vi "UI_WindowFrame.vi"(8 "error in (no error)":errorcluster, 11 "WindowFrame in":refnum<class "WindowFrame.lvclass">) -> (0 "error out":errorcluster, 3 "WindowFrame out":refnum<class "WindowFrame.lvclass">)   [LabVIEW 2025, in "WindowFrame.lvlib" / "WindowFrame.lvclass"]
uses:
  WindowFrame.lvclass
  C:/GitHub/danyallard/ClassUtilities/src/ClassByRef/ClassByRef.lvclass
  ClassUtilities/src/ClassByRef/ClassByRef.lvclass/ClassByRef.ctl
  <vilib>/event_ctls.llb/usereventprio.ctl
  Action.ctl
  <vilib>/Utility/miscctls.llb/LVPointTypeDef.ctl
  <vilib>/Utility/miscctls.llb/LVRectTypeDef.ctl
  FrontPanel.Open.ctl
  FrontPanel.Run-TimePosition.Centered.ctl
  FrontPanel.Run-TimePosition.Custom.ctl
  FrontPanel.Run-TimePosition.GetPosition.ctl
  SubPanelInfo.ctl
  <vilib>/Utility/miscctls.llb/LVPositionTypeDef.ctl
  <vilib>/Utility/miscctls.llb/LVBoundsTypeDef.ctl
  947dc2d2-893a-4bb1-96e4-45aff6c94e7a.vi
  ClassUtilities/src/ClassByRef/GetExitEvent.vi
  ClassUtilities/src/ClassByRef/GetNotifier.vi
  ClassUtilities/src/ClassByRef/GetExitEvent.vi/d78f5ac1-b881-48f7-a86d-8a9fda2b8e49.vi
  ClassUtilities/src/ClassByRef/GetNotifier.vi/815770e3-f244-4544-877a-43bf45f14863.vi
  ClassUtilities/src/ClassByRef/GetRef.vi
  GetEventActionRef.vi
  GetEventCloseRef.vi
  GetEventStateRef.vi
  ClassUtilities/src/ClassByRef/ClassByRef.lvclass
panel:
  in  "Close":bool
  in  "Maximize":bool
  in  "Minimize":bool
  out "TitleBar":bool=TRUE
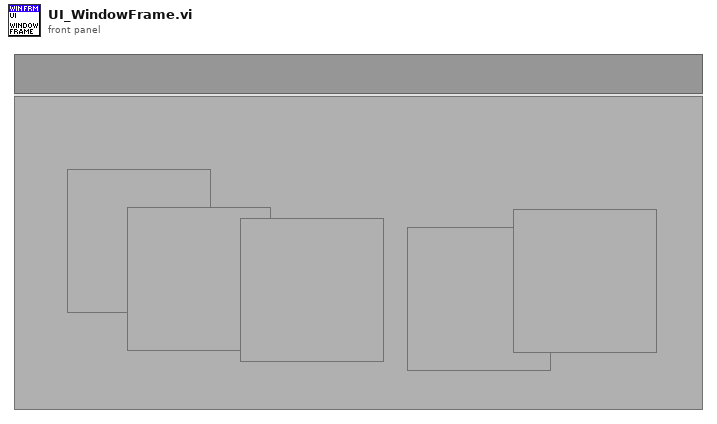
[diagram p1: front panel]
types:
  T1 = typedef "usereventprio.ctl" = enum32{"high priority", "normal priority"}
  T2 = enum32{"Invalid", "Standard", "Closed", "Hidden", "Minimized", "Maximized"}
  T3 = enum32{"Invalid", "Default", "Floating", "Floating/Auto-Hide", "Modal"}
  T4 = enum8{"Enabled", "Disabled", "Disabled and Grayed Out"}
  T5 = typedef "LVPointTypeDef.ctl" = cluster{"Horizontal":i16, "Vertical":i16}
  T6 = typedef "LVRectTypeDef.ctl" = cluster{"Left":i16, "Top":i16, "Right":i16, "Bottom":i16}
  T7 = typedef "WindowFrame.lvlib/WindowFrame.lvclass/FrontPanel.Open.ctl" = cluster{"Activate?":bool, "State":enum32{"Invalid", "Standard", "Closed", "Hidden", "Minimized", "Maximized"}}
  T8 = typedef "WindowFrame.lvlib/WindowFrame.lvclass/FrontPanel.Run-TimePosition.Centered.ctl" = cluster{"Monitor":i16, "Size":cluster{"Height":i16, "Width":i16}}
  T9 = typedef "WindowFrame.lvlib/WindowFrame.lvclass/FrontPanel.Run-TimePosition.Custom.ctl" = cluster{"Position":cluster{"Top":i16, "Left":i16}, "Size":cluster{"Height":i16, "Width":i16}}
  T10 = typedef "WindowFrame.lvlib/WindowFrame.lvclass/FrontPanel.Run-TimePosition.GetPosition.ctl" = cluster{"Type":enum32{"Unchanged", "Centered", "Maximized", "Minimized", "Custom"}, "Position":cluster{"Top":i16, "Left":i16}, "Size":cluster{"Height":i16, "Width":i16}, "Monitor":i16, "Use Current Position":bool, "Use Current Size":bool}
  T11 = typedef "WindowFrame.lvlib/WindowFrame.lvclass/SubPanelInfo.ctl" = cluster{"Z-Order":i32, "Position":T12, "Size":T13, "VI Ref":refnum<vi>}
  T12 = typedef "LVPositionTypeDef.ctl" = cluster{"Left":i32, "Top":i32}
  T13 = typedef "LVBoundsTypeDef.ctl" = cluster{"Width":u32, "Height":u32}
  T14 = cluster{"Event Registration Refnum":refnum<event-registration>}
  T15 = typedef "WindowFrame.lvlib/WindowFrame.lvclass/Action.ctl" = enum16{"Set Allow Runtime PopUp", "Set Behavior", "Set Closable", "Set Custom Title", "Set Highlight Return Button", "Set Is Frontmost", "Set Minimizable", "Set Minimum Size", "Set Monitor", "Set Resizable", "Set Panel Bounds", "Set Run VI Transparently", "Set Show Menu Bar", "Set State", "Set Title", "Set Title Bar Colors", "Set Title Bar Visible", "Set Transparancy", "Set Window Bounds", "Get Allow Runtime PopUp", "Get Behavior", "Get Closable", "Get Custom Title", "Get Highlight Return Button", "Get Is Frontmost", "Get Minimizable", "Get Minimum Size", "Get Monitor", "Get Panel Bounds", "Get Resizable", "Get Run VI Transparently", "Get Show Menu Bar", "Get State", "Get Title", "Get Title Bar Colors", "Get Title Bar Visible", "Get Transparancy", "Get Window Bounds", "--", "Center", "Close", "Open", "Run-Time Position:Centered", "Run-Time Position:Custom", "Run-Time Position:Get Position", "Run-Time Position:Maximized", "Run-Time Position:Minimized", "Run-Time Position:Unchanged", "---", "Insert VI", "Remove VI", "Insert VI Index", "Remove VI Index", "Exit"}
  T16 = enum32{"Unchanged", "Centered", "Maximized", "Minimized", "Custom"}
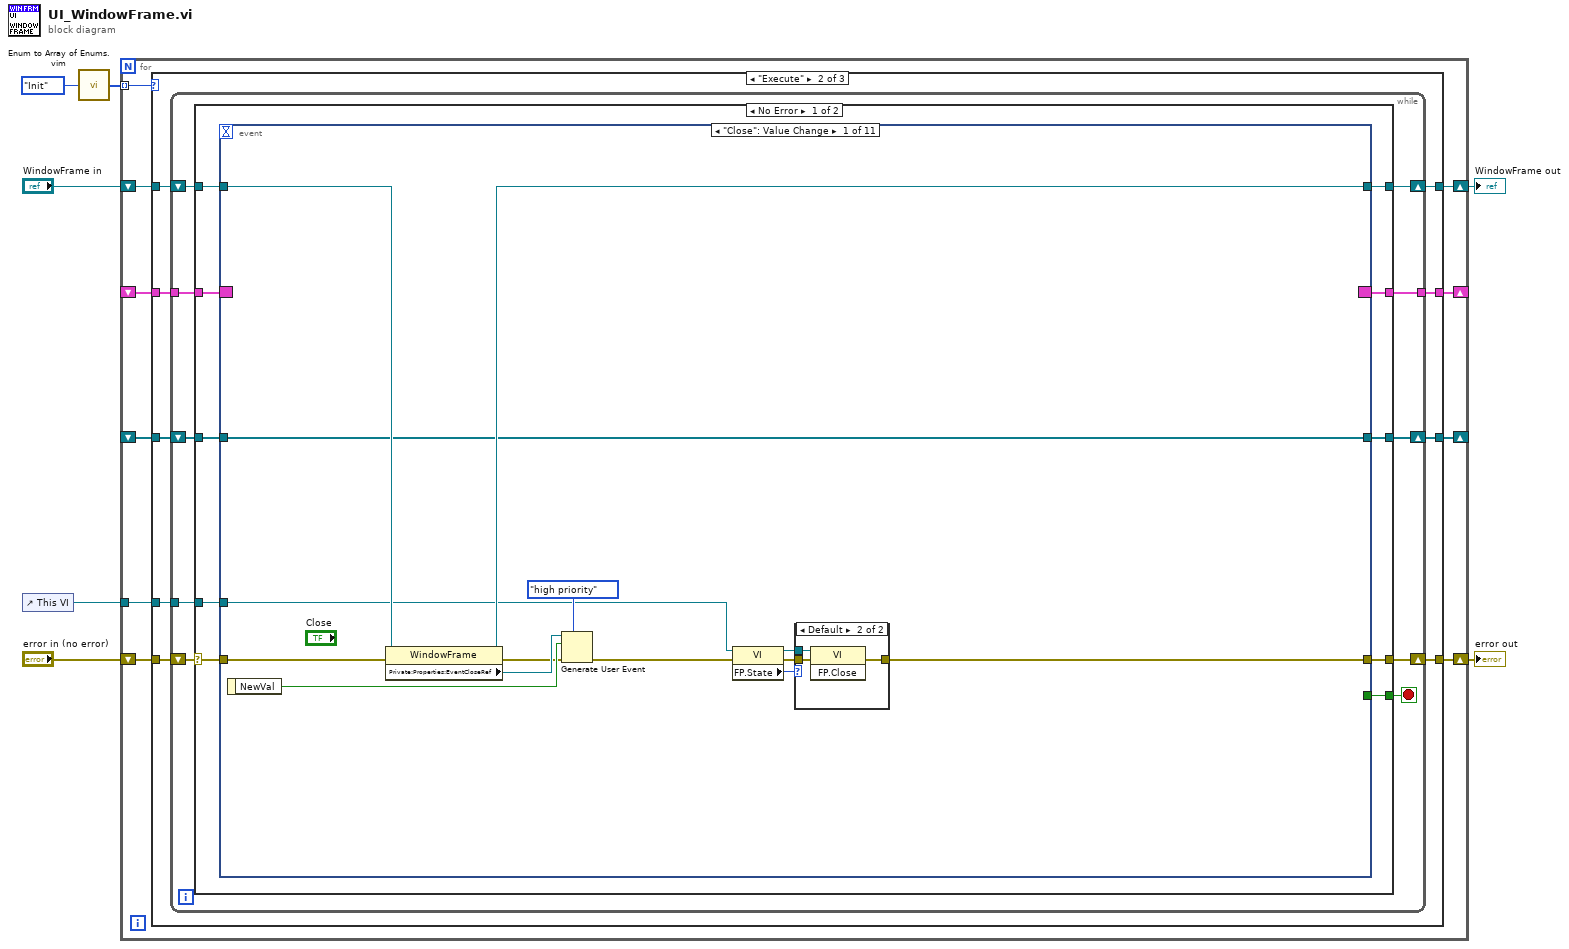
[diagram p0: block diagram]
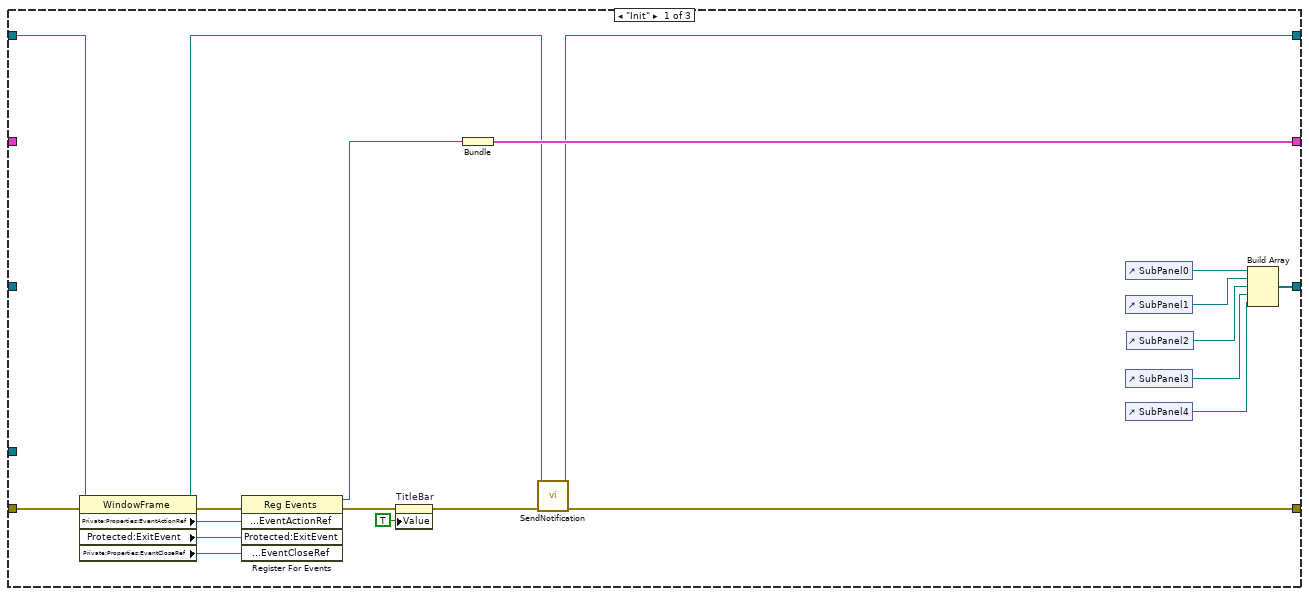
[diagram p2: hidden frame]
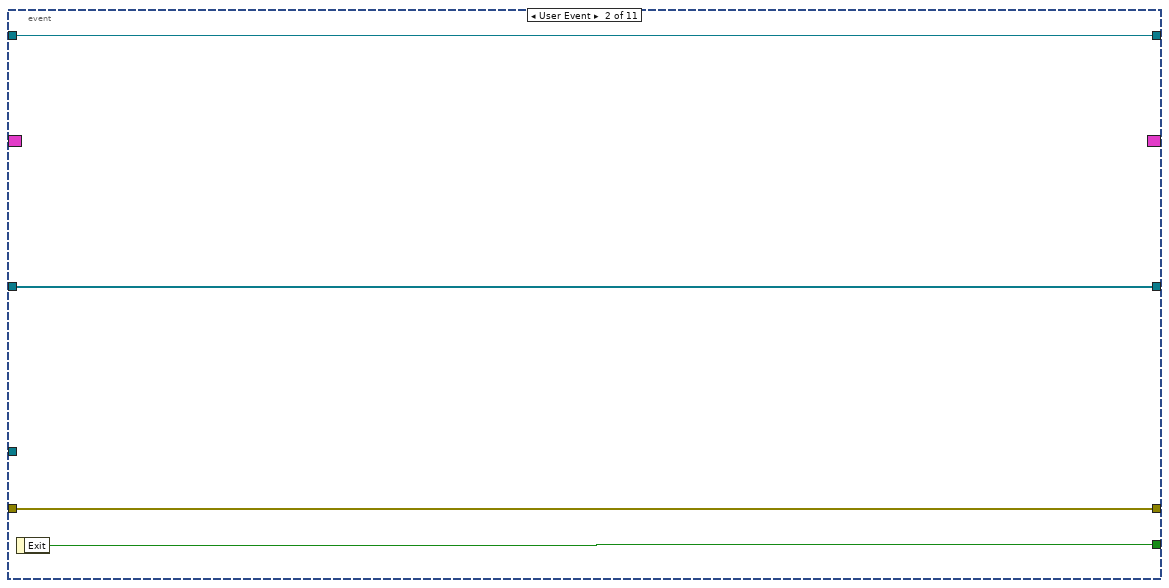
[diagram p4: hidden frame]
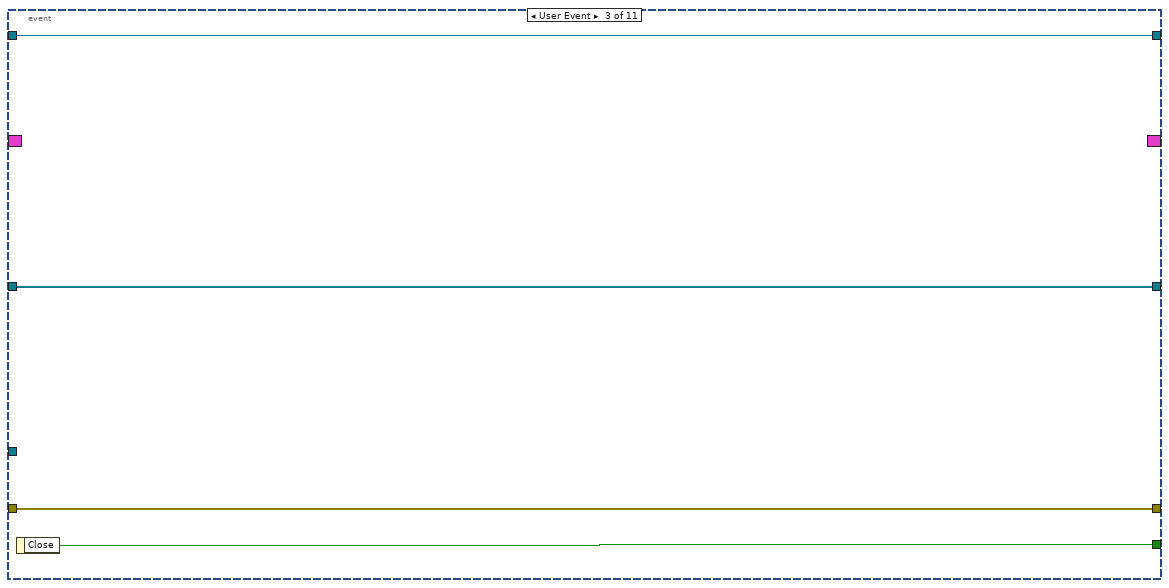
[diagram p5: hidden frame]
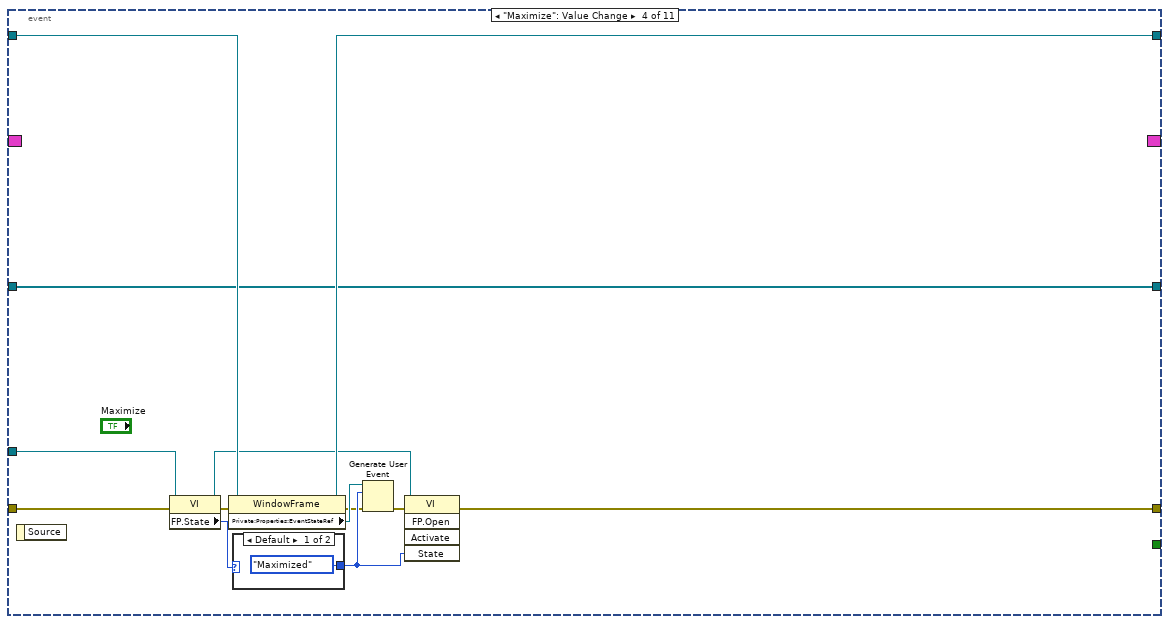
[diagram p6: hidden frame]
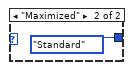
[diagram p7: hidden frame]
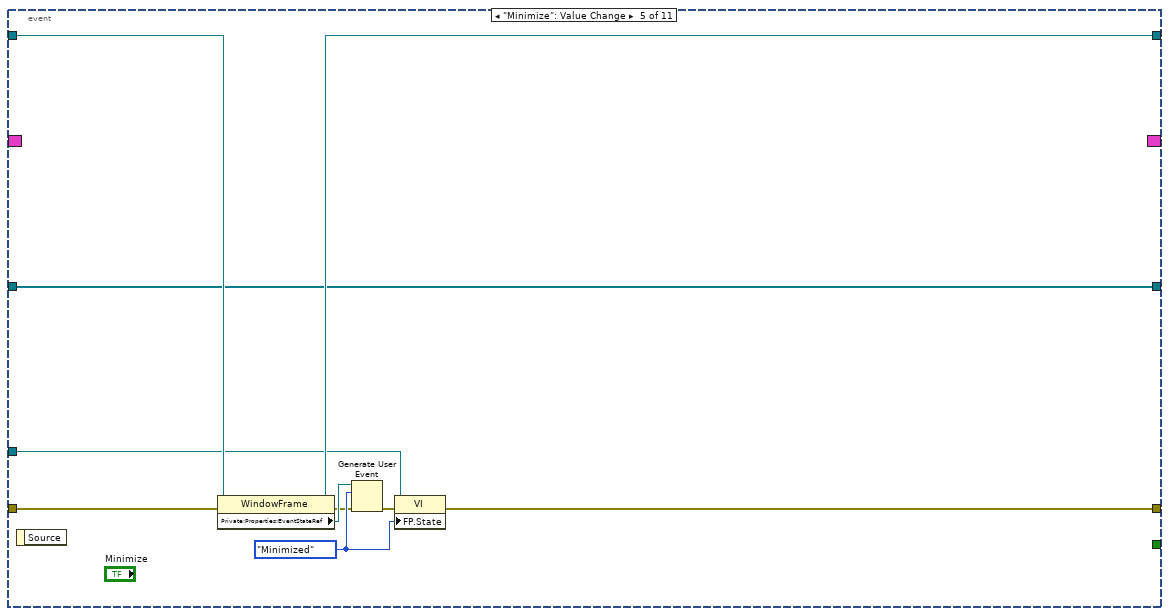
[diagram p8: hidden frame]
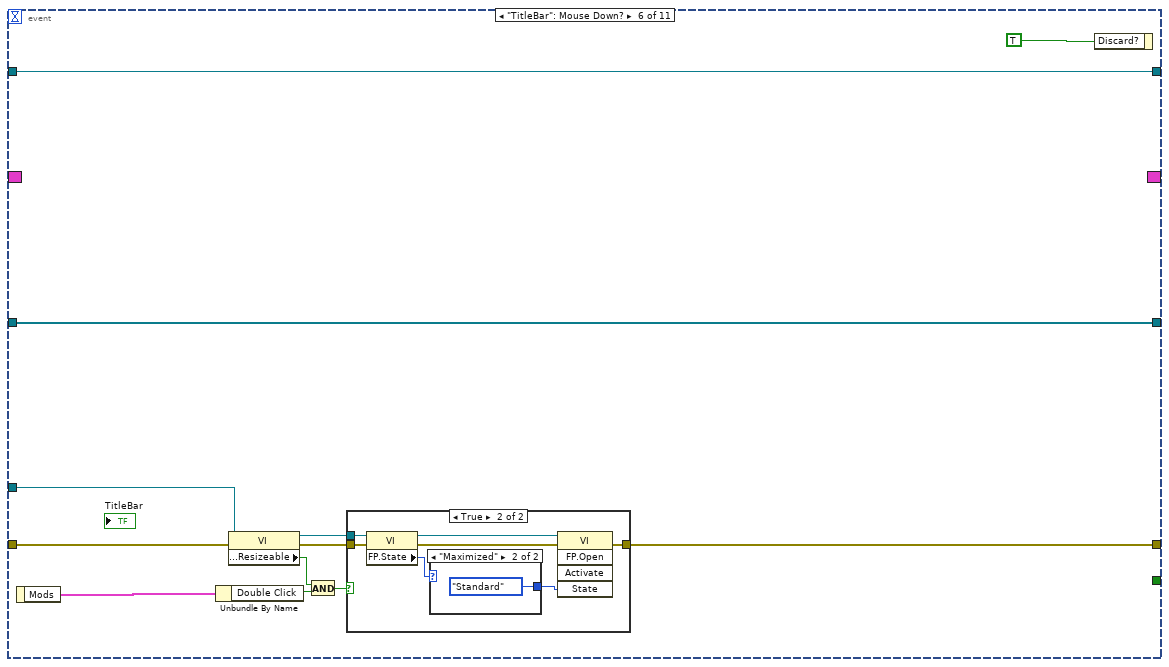
[diagram p9: hidden frame]
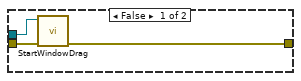
[diagram p10: hidden frame]
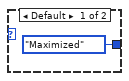
[diagram p11: hidden frame]
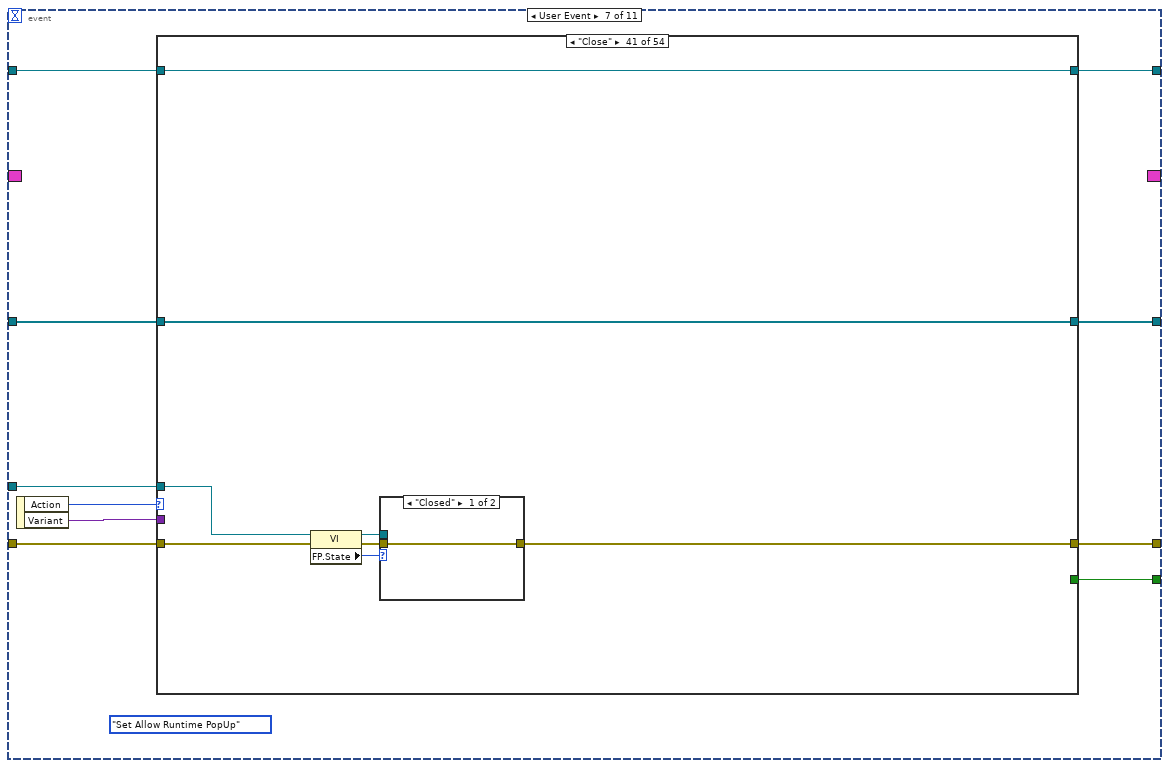
[diagram p12: hidden frame]
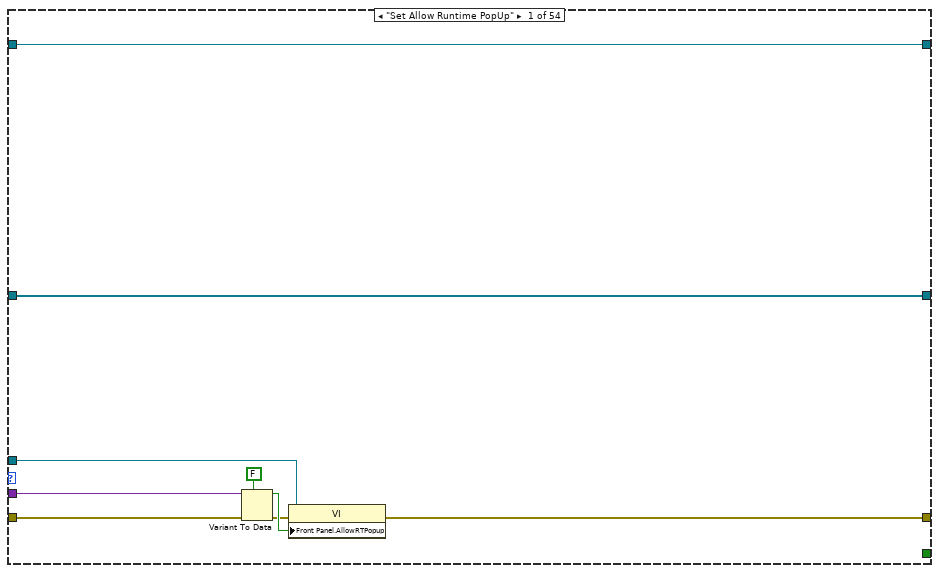
[diagram p13: hidden frame]
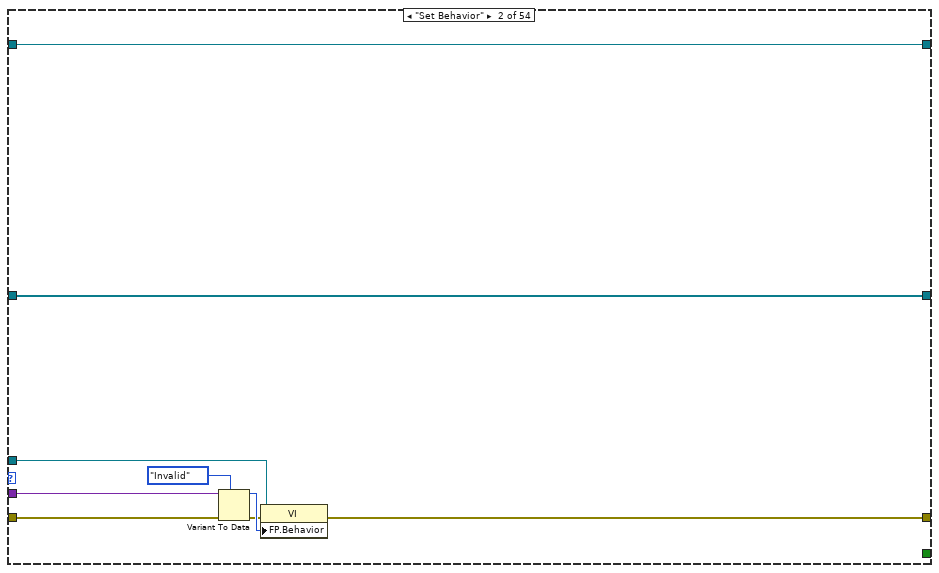
[diagram p14: hidden frame]
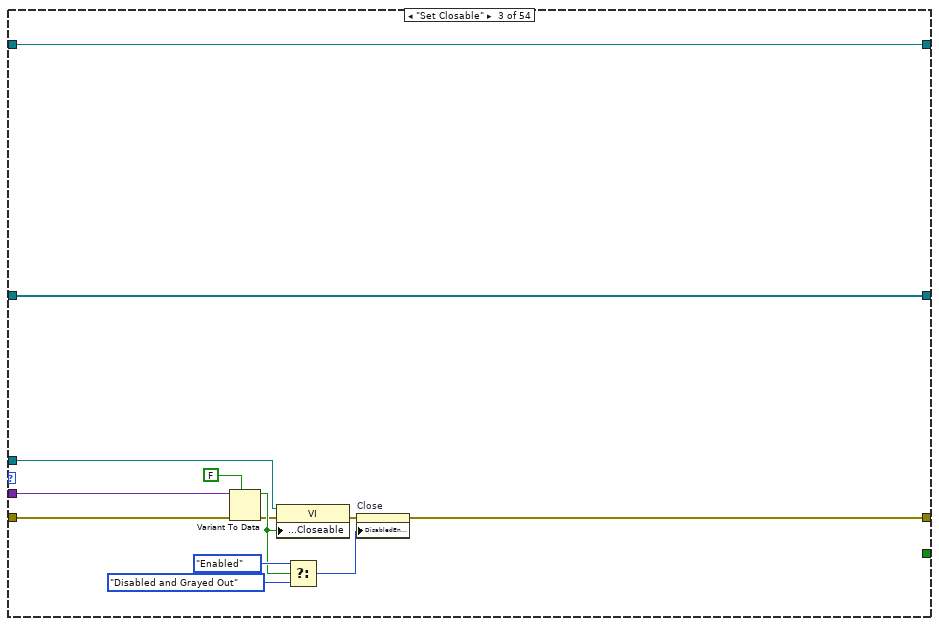
[diagram p15: hidden frame]
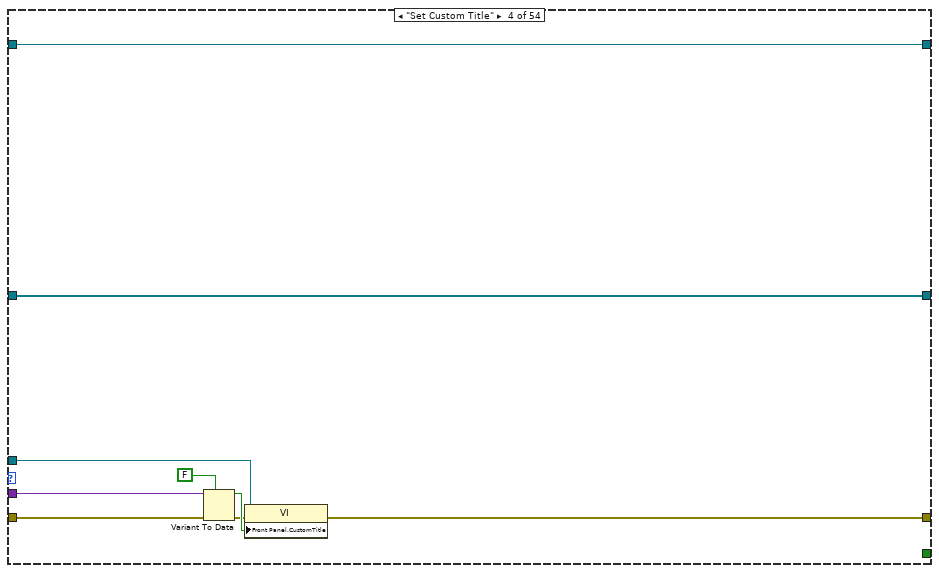
[diagram p16: hidden frame]
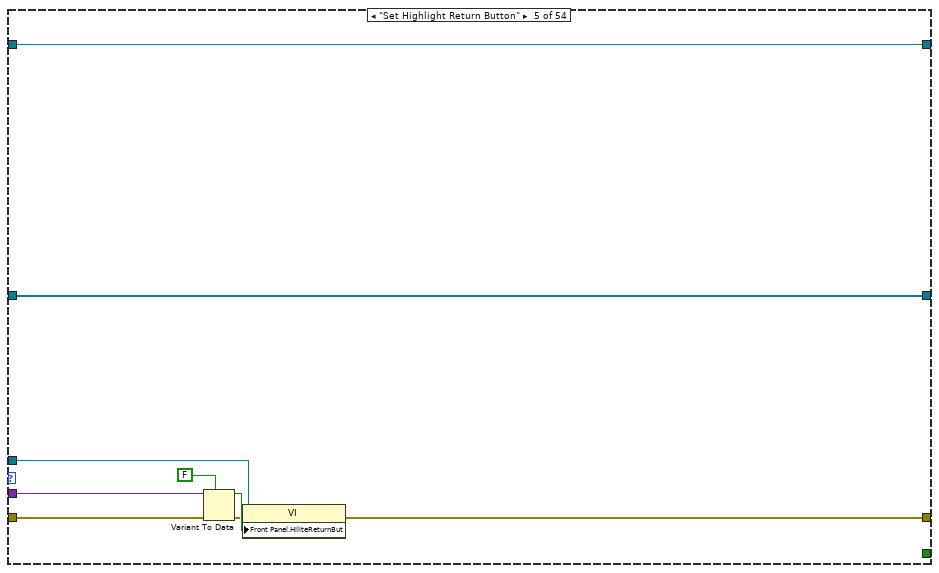
[diagram p17: hidden frame]
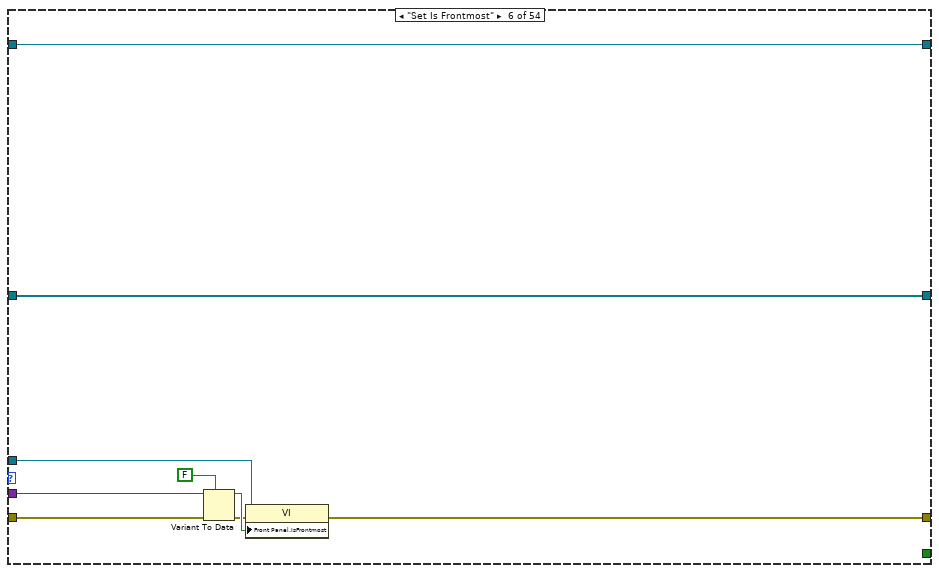
[diagram p18: hidden frame]
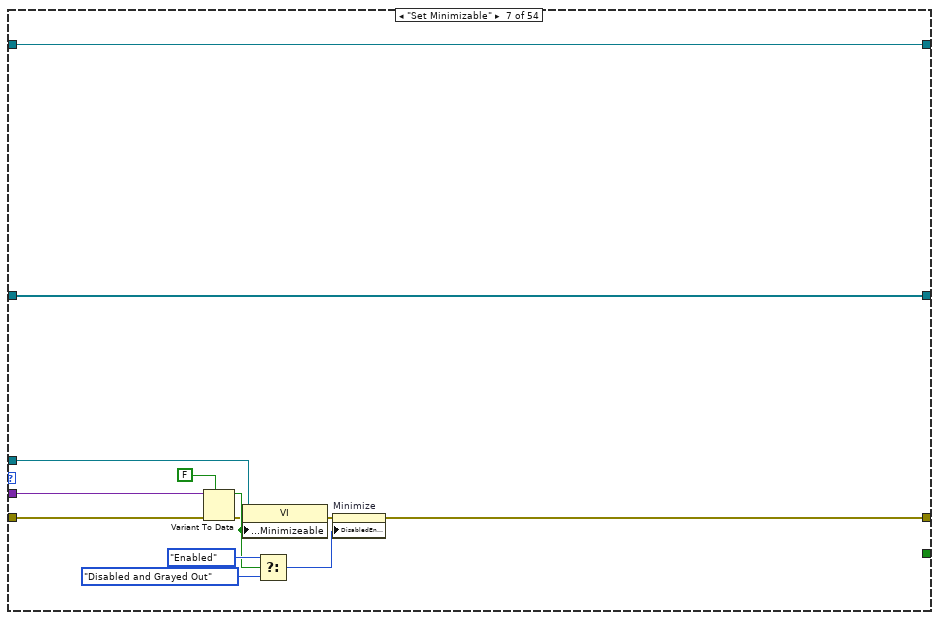
[diagram p19: hidden frame]
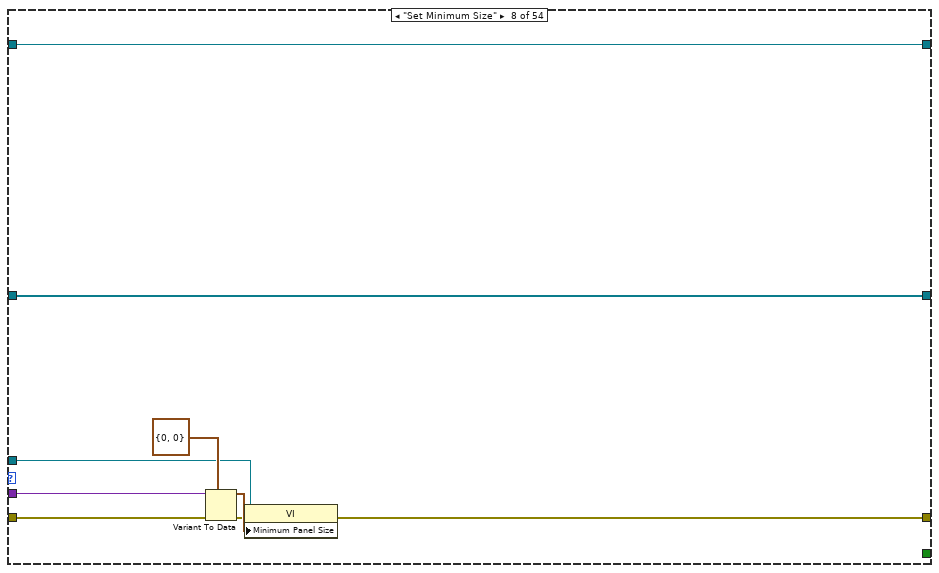
[diagram p20: hidden frame]
diagram:
  n1 = control-ref of="This VI"() -> (w6:refnum<vi>)
  n2 = call "Enum to Array of Enums.vim"("enum"=enum16{"Init", "Execute", "Close"}."Init") -> ("array of enums"=w4:enum16{"Init", "Execute", "Close"}[])
  n3 = for {
    tunnel: w6 -> [w15]
    shift-right: [w17] -> w7
    shift-left: "WindowFrame in" -> [w16]
    shift-right: [w9] -> _
    shift-left: _ -> [w14]
    shift-right: [w10] -> w3
    shift-left: "error in (no error)" -> [w13]
    tunnel: w4 -> [w11] mode=indexing
    shift-right: [w8] -> _
    shift-left: _ -> [w12]
    n4 = case shown="\"Execute\"" w11 {
      tunnel: [w22 w46 w785] -> w17
      tunnel: [w24 w45 w786] -> w10
      tunnel: w16 -> [w21 w44 w784]
      tunnel: w15 -> [_ w43 _]
      tunnel: w14 -> [_ w42 w790]
      tunnel: w13 -> [w27 w41 w789]
      tunnel: [w25 w40 w790] -> w9
      tunnel: w12 -> [_ w39 w787]
      tunnel: [w32 w38 w787] -> w8
      frame "Init" {
        n5 = property class="WindowFrame"(reference=w21, error in=w27) -> (reference out=w23:refnum<class "WindowFrame.lvclass">, error out=w30:errorcluster, "Private:Properties:EventActionRef"=w29:refnum<user-event>, "Protected:ExitEvent"=w19:refnum<user-event>, "Private:Properties:EventCloseRef"=w18:refnum<user-event>)
        n6 = register-events(error in=w30, w29, w19, w18) -> (reference out=w26:refnum<event-registration>, error out=w31:errorcluster)  [unwired: 1 in]
        n7 = property on="TitleBar" class="Bool (strict)"(error in=w31, "Value"=TRUE ("TitleBar")) -> (error out=w20:errorcluster)  [unwired: 1 in, 1 out]
        n8 = Bundle("Event Registration Refnum"=w26) -> (w25:T14)  [unwired: 1 in]
        n9 = call "SendNotification.vi"("error in (no error)"=w20, "ByRefClass in"=w23) -> ("error out"=w24:errorcluster, "ByRefClass out"=w22:refnum<class "WindowFrame.lvclass">)  [unwired: 8 in]
        n10 = control-ref of="SubPanel0"() -> (w34:refnum<vi>)
        n11 = control-ref of="SubPanel1"() -> (w33:refnum<vi>)
        n12 = control-ref of="SubPanel3"() -> (w36:refnum<vi>)
        n13 = control-ref of="SubPanel4"() -> (w37:refnum<vi>)
        n14 = control-ref of="SubPanel2"() -> (w35:refnum<vi>)
        n15 = Build Array(w34, w33, w35, w36, w37) -> (w32:refnum<vi>[])
      }
      frame "Execute" {
        n16 = while {
          shift-right: [w53] -> w46
          shift-left: w44 -> [w55]
          shift-right: [w54] -> w45
          shift-left: w41 -> [w51]
          tunnel: w43 -> [w52]
          tunnel: [w50] -> w40
          tunnel: w42 -> [w49]
          shift-right: [w47] -> w38
          shift-left: w39 -> [w48]
          stop <- w56 stop-if-true
          n17 = case shown="No Error" w51 {
            selector: w51 -> [w60 w783]
            tunnel: [w66 _] -> w56
            tunnel: w55 -> [w65 w780]
            tunnel: [w64 w781] -> w54
            tunnel: w49 -> [w63 w779]
            tunnel: [w62 w780] -> w53
            tunnel: w52 -> [w61 _]
            tunnel: [w59 w779] -> w50
            tunnel: w48 -> [w58 w778]
            tunnel: [w57 w778] -> w47
            frame No Error {
              n18 = event shown="[0] \"Close\": Value Change" {
                selector: w63 -> [_ _ _ _ _ _ _ _ _ _ _]
                dyn-events: [_ _ _ _ _ _ _ _ _ _ _] -> w59
                timeout: _ -> [_ _ _ _ _ _ _ _ _ _ _]
                tunnel: [_ w85 w89 _ _ _ w144 _ w754 _ _] -> w66
                tunnel: [w74 w88 w92 w98 w117 w123 w147 w751 w753 w759 w775] -> w64
                tunnel: w65 -> [w80 w87 w91 w104 w116 w119 w149 w750 w755 w763 w774]
                tunnel: [w75 w87 w91 w96 w111 w119 w146 w750 w755 w763 w774] -> w62
                tunnel: w60 -> [w72 w88 w92 w97 w112 w122 w148 w751 w753 w758 w775]
                tunnel: w61 -> [w70 _ _ w95 w109 w120 w145 _ _ w757 _]
                tunnel: w58 -> [w67 w86 w90 w93 w108 w118 w143 w746 w752 w756 w773]
                tunnel: [w67 w86 w90 w93 w108 w118 w142 w746 w752 w756 w773] -> w57
                event "Close": Value Change {
                  n19 = event-data() -> ("NewVal"=w78:bool)  [unwired: 1 in]
                  n20 = property class="WindowFrame"(reference=w80, error in=w72) -> (reference out=w75:refnum<class "WindowFrame.lvclass">, error out=w73:errorcluster, "Private:Properties:EventCloseRef"=w79:refnum<user-event>)
                  n21 = Generate User Event(priority (normal)=usereventprio."high priority", user event=w79, event data cluster=w78, error in=w73) -> (error out=w76:errorcluster)  [unwired: 1 out]
                  n22 = property class="VI"(reference=w70, error in=w76) -> (reference out=w69:refnum<vi>, error out=w71:errorcluster, "FP.State"=w68:T2)
                  n23 = case shown="Default" w68 {
                    tunnel: [w81 w84] -> w74
                    tunnel: w71 -> [w81 w83]
                    tunnel: w69 -> [_ w82]
                    frame "Closed" {
                    }
                    frame Default {
                      n24 = invoke class="VI" method="FP.Close"(reference=w82, error in=w83) -> (error out=w84:errorcluster)  [unwired: 1 in, 2 out]
                    }
                  }
                }
                event User Event {
                  n25 = event-data() -> ("Exit"=w85:bool)  [unwired: 1 in]
                }
                event User Event {
                  n26 = event-data() -> ("Close"=w89:bool)  [unwired: 1 in]
                }
                event "Maximize": Value Change {
                  n27 = event-data() -> ()  [unwired: 1 in, 1 out]
                  n28 = property class="VI"(reference=w95, error in=w97) -> (reference out=w94:refnum<vi>, error out=w101:errorcluster, "FP.State"=w105:T2)
                  n29 = property class="WindowFrame"(reference=w104, error in=w101) -> (reference out=w96:refnum<class "WindowFrame.lvclass">, error out=w100:errorcluster, "Private:Properties:EventStateRef"=w103:refnum<user-event>)
                  n30 = case shown="Default" w105 {
                    tunnel: [T2."Maximized" ("State") T2."Standard" ("State")] -> w102
                    frame Default {
                    }
                    frame "Maximized" {
                    }
                  }
                  n31 = Generate User Event(user event=w103, event data cluster=w102, error in=w100) -> (error out=w99:errorcluster)  [unwired: 1 in, 1 out]
                  n32 = invoke class="VI" method="FP.Open"(reference=w94, error in=w99, "State"=w102) -> (error out=w98:errorcluster)  [unwired: 2 in, 4 out]
                }
                event "Minimize": Value Change {
                  w114 = T2."Minimized" ("State")
                  n33 = event-data() -> ()  [unwired: 1 in, 1 out]
                  n34 = property class="WindowFrame"(reference=w116, error in=w112) -> (reference out=w111:refnum<class "WindowFrame.lvclass">, error out=w110:errorcluster, "Private:Properties:EventStateRef"=w115:refnum<user-event>)
                  n35 = Generate User Event(user event=w115, event data cluster=w114, error in=w110) -> (error out=w113:errorcluster)  [unwired: 1 in, 1 out]
                  n36 = property class="VI"(reference=w109, error in=w113, "FP.State"=w114) -> (error out=w117:errorcluster)  [unwired: 1 out]
                }
                event "TitleBar": Mouse Down? {
                  n37 = event-data() -> ("Mods"=w128:cluster{"Double Click":bool, "Menu Key":bool})  [unwired: 1 in]
                  n38 = Unbundle By Name(w128) -> ("Double Click"=w127:bool)
                  n39 = property class="VI"(reference=w120, error in=w122) -> (reference out=w121:refnum<vi>, error out=w124:errorcluster, "Front Panel.Resizeable"=w125:bool)
                  n40 = And(x=w125, y=w127) -> (x .and. y?=w126:bool)
                  n41 = case shown="True" w126 {
                    tunnel: w124 -> [w132 w137]
                    tunnel: [w131 w135] -> w123
                    tunnel: w121 -> [w130 w134]
                    frame False {
                      n42 = call "StartWindowDrag.vi"("error in (no error)"=w132, "VI Ref (calling VI)"=w130) -> ("error out"=w131:errorcluster)  [unwired: 8 in, 1 out]
                    }
                    frame True {
                      n43 = property class="VI"(reference=w134, error in=w137) -> (reference out=w133:refnum<vi>, error out=w136:errorcluster, "FP.State"=w138:T2)
                      n44 = case shown="\"Maximized\"" w138 {
                        tunnel: [T2."Maximized" ("State") T2."Standard" ("State")] -> w139
                        frame Default {
                        }
                        frame "Maximized" {
                        }
                      }
                      n45 = invoke class="VI" method="FP.Open"(reference=w133, error in=w136, "State"=w139) -> (error out=w135:errorcluster)  [unwired: 2 in, 4 out]
                    }
                  }
                  n46 = event-data("Discard?"=TRUE) -> ()  [unwired: 1 in, 1 out]
                }
                event User Event {
                  (unwired) Action."Set Allow Runtime PopUp" ("Action")
                  n47 = event-data() -> ("Action"=w151:T15, "Variant"=w150:variant)  [unwired: 1 in]
                  n48 = case shown="\"Close\"" w151 {
                    tunnel: w150 -> [w160 w169 w182 w191 w200 w209 w222 w231 w240 w249 w262 w271 w279 w288 w301 w321 w341 w350 w359 w370 w381 w392 w403 w414 w425 w436 w448 w459 w470 w481 w492 w503 w514 w525 w536 w546 w557 w568 _ _ _ w600 w620 w658 w668 w684 w693 _ _ w707 w722 w735 _ _]
                    tunnel: w149 -> [w154 w166 w177 w188 w197 w207 w217 w228 w238 w246 w257 w269 w277 w285 w296 w319 w339 w348 w356 w367 w378 w389 w400 w411 w422 w433 w445 w456 w467 w478 w489 w500 w511 w522 w533 w543 w554 w565 w570 w575 w583 w589 w616 w653 w664 w682 w691 w698 w700 w709 w724 w737 w741 w744]
                    tunnel: w148 -> [w155 w163 w173 w184 w194 w204 w213 w225 w235 w243 w253 w266 w274 w282 w292 w316 w334 w345 w353 w363 w374 w385 w396 w407 w418 w429 w441 w452 w463 w474 w485 w496 w507 w518 w529 w541 w550 w561 w571 w573 w581 w594 w613 w650 w660 w679 w688 w696 w701 w708 w723 w736 w740 w745]
                    tunnel: [w156 w164 w174 w185 w195 w205 w214 w226 w236 w244 w254 w267 w275 w283 w293 w317 w332 w346 w354 w364 w375 w386 w397 w408 w419 w430 w442 w453 w464 w475 w486 w497 w508 w519 w530 w542 w551 w562 w571 w574 w582 w590 w614 w651 w661 w680 w689 w697 w701 w705 w716 w732 w739 w745] -> w147
                    tunnel: [w154 w166 w177 w188 w197 w207 w217 w228 w238 w246 w257 w269 w277 w285 w296 w319 w339 w348 w356 w367 w378 w389 w400 w411 w422 w433 w445 w456 w467 w478 w489 w500 w511 w522 w533 w543 w554 w565 w570 w575 w583 w588 w616 w653 w664 w682 w691 w698 w700 w709 w724 w737 w741 w744] -> w146
                    tunnel: w145 -> [w153 w162 w171 w186 w193 w203 w212 w224 w233 w242 w252 w264 _ w281 w291 _ w326 w343 w352 w362 w373 w384 w395 w406 w417 w428 w440 w451 w462 w473 w484 w495 w506 w517 w528 _ w549 w560 _ _ w579 w593 w611 w649 _ w677 w686 w695 _ w702 _ _ _ _]
                    tunnel: [_ _ _ _ _ _ _ _ _ _ _ _ _ _ _ _ _ _ _ _ _ _ _ _ _ _ _ _ _ _ _ _ _ _ _ _ _ _ _ _ _ _ _ _ _ _ _ _ _ _ _ _ _ TRUE] -> w144
                    tunnel: w143 -> [w152 w161 w170 w183 w192 w201 w210 w223 w232 w241 w250 w263 w272 w280 w289 w314 w322 w342 w351 w360 w371 w382 w393 w404 w415 w426 w437 w449 w460 w471 w482 w493 w504 w515 w526 w537 w547 w558 w569 w572 w576 w591 w610 w648 w659 w676 w685 w694 w699 w703 w710 w725 w738 w742]
                    tunnel: [w152 w161 w170 w183 w192 w201 w210 w223 w232 w241 w250 w263 w272 w280 w289 w314 w322 w342 w351 w360 w371 w382 w393 w404 w415 w426 w437 w449 w460 w471 w482 w493 w504 w515 w526 w537 w547 w558 w569 w572 w576 w591 w610 w648 w659 w676 w685 w694 w699 w703 w710 w725 w738 w742] -> w142
                    frame "Set Allow Runtime PopUp" {
                      n49 = Variant To Data(error in=w155, type=FALSE, Variant=w160) -> (data=w158:bool, error out=w157:errorcluster)
                      n50 = property class="VI"(reference=w153, error in=w157, "Front Panel.AllowRTPopup"=w158) -> (error out=w156:errorcluster)  [unwired: 1 out]
                    }
                    frame "Set Behavior" {
                      n51 = Variant To Data(error in=w163, type=T3."Invalid" ("Front Panel Window:Behavior"), Variant=w169) -> (data=w167:T3, error out=w165:errorcluster)
                      n52 = property class="VI"(reference=w162, error in=w165, "FP.Behavior"=w167) -> (error out=w164:errorcluster)  [unwired: 1 out]
                    }
                    frame "Set Closable" {
                      n53 = Variant To Data(error in=w173, type=FALSE, Variant=w182) -> (data=w179:bool, error out=w176:errorcluster)
                      n54 = property class="VI"(reference=w171, error in=w176, "Front Panel.Closeable"=w179) -> (error out=w175:errorcluster)  [unwired: 1 out]
                      n55 = Select(t=T4."Enabled" ("Disabled"), s=w179, f=T4."Disabled and Grayed Out" ("Disabled")) -> (s? t:f=w178:T4)
                      n56 = property on="Close" class="Bool"(error in=w175, "DisabledEnum"=w178) -> (error out=w174:errorcluster)  [unwired: 1 in, 1 out]
                    }
                    frame "Set Custom Title" {
                      n57 = Variant To Data(error in=w184, type=FALSE, Variant=w191) -> (data=w189:bool, error out=w187:errorcluster)
                      n58 = property class="VI"(reference=w186, error in=w187, "Front Panel.CustomTitle"=w189) -> (error out=w185:errorcluster)  [unwired: 1 out]
                    }
                    frame "Set Highlight Return Button" {
                      n59 = Variant To Data(error in=w194, type=FALSE, Variant=w200) -> (data=w198:bool, error out=w196:errorcluster)
                      n60 = property class="VI"(reference=w193, error in=w196, "Front Panel.HiliteReturnBut"=w198) -> (error out=w195:errorcluster)  [unwired: 1 out]
                    }
                    frame "Set Is Frontmost" {
                      n61 = Variant To Data(error in=w204, type=FALSE, Variant=w209) -> (data=w208:bool, error out=w206:errorcluster)
                      n62 = property class="VI"(reference=w203, error in=w206, "Front Panel.IsFrontmost"=w208) -> (error out=w205:errorcluster)  [unwired: 1 out]
                    }
                    frame "Set Minimizable" {
                      n63 = Variant To Data(error in=w213, type=FALSE, Variant=w222) -> (data=w219:bool, error out=w216:errorcluster)
                      n64 = property class="VI"(reference=w212, error in=w216, "Front Panel.Minimizeable"=w219) -> (error out=w215:errorcluster)  [unwired: 1 out]
                      n65 = Select(t=T4."Enabled" ("Disabled"), s=w219, f=T4."Disabled and Grayed Out" ("Disabled")) -> (s? t:f=w218:T4)
                      n66 = property on="Minimize" class="Bool"(error in=w215, "DisabledEnum"=w218) -> (error out=w214:errorcluster)  [unwired: 1 in, 1 out]
                    }
                    frame "Set Minimum Size" {
                      n67 = Variant To Data(error in=w225, type=T5 {"Horizontal"=0, "Vertical"=0} ("Front Panel Window:Minimum Size"), Variant=w231) -> (data=w229:T5, error out=w227:errorcluster)
                      n68 = property class="VI"(reference=w224, error in=w227, "Minimum Panel Size"=w229) -> (error out=w226:errorcluster)  [unwired: 1 out]
                    }
                    frame "Set Monitor" {
                      n69 = Variant To Data(error in=w235, type=u16 0 ("Front Panel Window:Monitor"), Variant=w240) -> (data=w239:u16, error out=w237:errorcluster)
                      n70 = property class="VI"(reference=w233, error in=w237, "FP.Monitor"=w239) -> (error out=w236:errorcluster)  [unwired: 1 out]
                    }
                    frame "Set Resizable" {
                      n71 = Variant To Data(error in=w243, type=T6 {"Left"=0, "Top"=0, "Right"=0, "Bottom"=0} ("Front Panel Window:Panel Bounds"), Variant=w249) -> (data=w247:T6, error out=w245:errorcluster)
                      n72 = property class="VI"(reference=w242, error in=w245, "Front Panel.PanelBounds"=w247) -> (error out=w244:errorcluster)  [unwired: 1 out]
                    }
                    frame "Set Panel Bounds" {
                      n73 = Variant To Data(error in=w253, type=FALSE, Variant=w262) -> (data=w258:bool, error out=w256:errorcluster)
                      n74 = property class="VI"(reference=w252, error in=w256, "Front Panel.Resizeable"=w258) -> (error out=w255:errorcluster)  [unwired: 1 out]
                      n75 = Select(t=T4."Enabled" ("Disabled"), s=w258, f=T4."Disabled and Grayed Out" ("Disabled")) -> (s? t:f=w259:T4)
                      n76 = property on="Maximize" class="Bool"(error in=w255, "DisabledEnum"=w259) -> (error out=w254:errorcluster)  [unwired: 1 in, 1 out]
                    }
                    frame "Set Run VI Transparently" {
                      n77 = Variant To Data(error in=w266, type=FALSE, Variant=w271) -> (data=w270:bool, error out=w268:errorcluster)
                      n78 = property class="VI"(reference=w264, error in=w268, "FP:RunTransparently"=w270) -> (error out=w267:errorcluster)  [unwired: 1 out]
                    }
                    frame "Set Show Menu Bar" {
                      n79 = Variant To Data(error in=w274, type=FALSE, Variant=w279) -> (data=w278:bool, error out=w276:errorcluster)
                      n80 = property class="VI"(error in=w276, "Front Panel.ShowMenuBar"=w278) -> (error out=w275:errorcluster)  [unwired: 1 in, 1 out]
                    }
                    frame "Set State" {
                      n81 = Variant To Data(error in=w282, type=T2."Invalid" ("Front Panel Window:State"), Variant=w288) -> (data=w287:T2, error out=w284:errorcluster)
                      n82 = property class="VI"(reference=w281, error in=w284, "FP.State"=w287) -> (error out=w283:errorcluster)  [unwired: 1 out]
                    }
                    frame "Set Title" {
                      n83 = Variant To Data(error in=w292, type="", Variant=w301) -> (data=w299:string, error out=w295:errorcluster)
                      n84 = property class="VI"(reference=w291, error in=w295) -> (reference out=w290:refnum<vi>, error out=w294:errorcluster, "Front Panel.CustomTitle"=w298:bool, "Front Panel.Title"=w297:string)
                      n85 = case shown="True" w298 {
                        tunnel: w299 -> [w304 _]
                        tunnel: w297 -> [_ w311]
                        tunnel: w294 -> [w308 w313]
                        tunnel: [w306 w312] -> w293
                        tunnel: w290 -> [w305 _]
                        frame True {
                          n86 = property class="VI"(reference=w305, error in=w308, "Front Panel.Title"=w304) -> (error out=w307:errorcluster)  [unwired: 1 out]
                          n87 = Initialize Array(w304, 4 ("dimension size")) -> (w303:string[])
                          n88 = property on="Title" class="Bool (strict)"(error in=w307, "Strings [4]"=w303) -> (error out=w306:errorcluster)  [unwired: 1 in, 1 out]
                        }
                        frame False {
                          n89 = Initialize Array(w311, 4 ("dimension size")) -> (w309:string[])
                          n90 = property on="Title" class="Bool (strict)"(error in=w313, "Strings [4]"=w309) -> (error out=w312:errorcluster)  [unwired: 1 in, 1 out]
                        }
                      }
                    }
                    frame "Set Title Bar Colors" {
                      n91 = Variant To Data(error in=w316, type=cluster{u32, u32}[] [{9868950, 9868950}, {13816530, 13816530}, {9868950, 9868950}, {13816530, 13816530}] ("Colors [4]"), Variant=w321) -> (data=w320:cluster{u32, u32}[], error out=w318:errorcluster)
                      n92 = property on="TitleBar" class="Bool (strict)"(error in=w318, "Colors [4]"=w320) -> (error out=w317:errorcluster)  [unwired: 1 in, 1 out]
                    }
                    frame "Set Title Bar Visible" {
                      n93 = Variant To Data(error in=w334, type=FALSE, Variant=w341) -> (data=w340:bool, error out=w338:errorcluster)
                      n94 = property class="VI"(reference=w326, error in=w338, "Front Panel.TitleBarVis"=w340) -> (error out=w337:errorcluster)  [unwired: 1 out]
                      n95 = Not(x=w340) -> (.not. x?=w331:bool)
                      n96 = property on="Minimize" class="Bool"(error in=w337, "Visible"=w331) -> (error out=w336:errorcluster)  [unwired: 1 in, 1 out]
                      n97 = property on="Maximize" class="Bool"(error in=w336, "Visible"=w331) -> (error out=w335:errorcluster)  [unwired: 1 in, 1 out]
                      n98 = property on="Close" class="Bool"(error in=w335, "Visible"=w331) -> (error out=w329:errorcluster)  [unwired: 1 in, 1 out]
                      n99 = property class="VI"(reference=w326, error in=w329) -> (error out=w328:errorcluster, "Front Panel.Title"=w327:string)  [unwired: 1 out]
                      n100 = Select(t=w327, s=w331, f="") -> (s? t:f=w325:string)
                      n101 = Initialize Array(w325, 4 ("dimension size")) -> (w324:string[])
                      n102 = property on="TitleBar" class="Bool (strict)"(error in=w328, "Strings [4]"=w324) -> (error out=w332:errorcluster)  [unwired: 1 in, 1 out]
                    }
                    frame "Set Transparancy" {
                      n103 = Variant To Data(error in=w345, type=u8 0 ("Front Panel Window:Transparency"), Variant=w350) -> (data=w349:u8, error out=w347:errorcluster)
                      n104 = property class="VI"(reference=w343, error in=w347, "FP:Transparency"=w349) -> (error out=w346:errorcluster)  [unwired: 1 out]
                    }
                    frame "Set Window Bounds" {
                      n105 = Variant To Data(error in=w353, type=T6 {"Left"=0, "Top"=0, "Right"=0, "Bottom"=0} ("Front Panel Window:Window Bounds"), Variant=w359) -> (data=w357:T6, error out=w355:errorcluster)
                      n106 = property class="VI"(reference=w352, error in=w355, "Front Panel.WinBounds"=w357) -> (error out=w354:errorcluster)  [unwired: 1 out]
                    }
                    frame "Get Allow Runtime PopUp" {
                      n107 = Variant To Data(error in=w363, type=refnum<notifier> refnum ("notifier out"), Variant=w370) -> (data=w369:refnum<notifier>, error out=w366:errorcluster)
                      n108 = property class="VI"(reference=w362, error in=w366) -> (error out=w365:errorcluster, "Front Panel.AllowRTPopup"=w361:bool)  [unwired: 1 out]
                      n109 = Send Notification(notification=w361, notifier=w369, error in (no error)=w365) -> (error out=w364:errorcluster)  [unwired: 1 out]
                    }
                    frame "Get Behavior" {
                      n110 = Variant To Data(error in=w374, type=refnum<notifier> refnum ("notifier out"), Variant=w381) -> (data=w380:refnum<notifier>, error out=w377:errorcluster)
                      n111 = property class="VI"(reference=w373, error in=w377) -> (error out=w376:errorcluster, "FP.Behavior"=w372:T3)  [unwired: 1 out]
                      n112 = Send Notification(notification=w372, notifier=w380, error in (no error)=w376) -> (error out=w375:errorcluster)  [unwired: 1 out]
                    }
                    frame "Get Closable" {
                      n113 = Variant To Data(error in=w385, type=refnum<notifier> refnum ("notifier out"), Variant=w392) -> (data=w391:refnum<notifier>, error out=w388:errorcluster)
                      n114 = property class="VI"(reference=w384, error in=w388) -> (error out=w387:errorcluster, "Front Panel.Closeable"=w383:bool)  [unwired: 1 out]
                      n115 = Send Notification(notification=w383, notifier=w391, error in (no error)=w387) -> (error out=w386:errorcluster)  [unwired: 1 out]
                    }
                    frame "Get Custom Title" {
                      n116 = Variant To Data(error in=w396, type=refnum<notifier> refnum ("notifier out"), Variant=w403) -> (data=w402:refnum<notifier>, error out=w399:errorcluster)
                      n117 = property class="VI"(reference=w395, error in=w399) -> (error out=w398:errorcluster, "Front Panel.CustomTitle"=w394:bool)  [unwired: 1 out]
                      n118 = Send Notification(notification=w394, notifier=w402, error in (no error)=w398) -> (error out=w397:errorcluster)  [unwired: 1 out]
                    }
                    frame "Get Highlight Return Button" {
                      n119 = Variant To Data(error in=w407, type=refnum<notifier> refnum ("notifier out"), Variant=w414) -> (data=w413:refnum<notifier>, error out=w410:errorcluster)
                      n120 = property class="VI"(reference=w406, error in=w410) -> (error out=w409:errorcluster, "Front Panel.HiliteReturnBut"=w405:bool)  [unwired: 1 out]
                      n121 = Send Notification(notification=w405, notifier=w413, error in (no error)=w409) -> (error out=w408:errorcluster)  [unwired: 1 out]
                    }
                    frame "Get Is Frontmost" {
                      n122 = Variant To Data(error in=w418, type=refnum<notifier> refnum ("notifier out"), Variant=w425) -> (data=w424:refnum<notifier>, error out=w421:errorcluster)
                      n123 = property class="VI"(reference=w417, error in=w421) -> (error out=w420:errorcluster, "Front Panel.IsFrontmost"=w416:bool)  [unwired: 1 out]
                      n124 = Send Notification(notification=w416, notifier=w424, error in (no error)=w420) -> (error out=w419:errorcluster)  [unwired: 1 out]
                    }
                    frame "Get Minimizable" {
                      n125 = Variant To Data(error in=w429, type=refnum<notifier> refnum ("notifier out"), Variant=w436) -> (data=w435:refnum<notifier>, error out=w432:errorcluster)
                      n126 = property class="VI"(reference=w428, error in=w432) -> (error out=w431:errorcluster, "Front Panel.Minimizeable"=w427:bool)  [unwired: 1 out]
                      n127 = Send Notification(notification=w427, notifier=w435, error in (no error)=w431) -> (error out=w430:errorcluster)  [unwired: 1 out]
                    }
                    frame "Get Minimum Size" {
                      n128 = Variant To Data(error in=w441, type=refnum<notifier> refnum ("notifier out"), Variant=w448) -> (data=w447:refnum<notifier>, error out=w444:errorcluster)
                      n129 = property class="VI"(reference=w440, error in=w444) -> (error out=w443:errorcluster, "Minimum Panel Size"=w439:T5)  [unwired: 1 out]
                      n130 = To Variant(anything=w439) -> (Variant=w438:variant)
                      n131 = Send Notification(notification=w438, notifier=w447, error in (no error)=w443) -> (error out=w442:errorcluster)  [unwired: 1 out]
                    }
                    frame "Get Monitor" {
                      n132 = Variant To Data(error in=w452, type=refnum<notifier> refnum ("notifier out"), Variant=w459) -> (data=w458:refnum<notifier>, error out=w455:errorcluster)
                      n133 = property class="VI"(reference=w451, error in=w455) -> (error out=w454:errorcluster, "FP.Monitor"=w450:u16)  [unwired: 1 out]
                      n134 = Send Notification(notification=w450, notifier=w458, error in (no error)=w454) -> (error out=w453:errorcluster)  [unwired: 1 out]
                    }
                    frame "Get Panel Bounds" {
                      n135 = Variant To Data(error in=w463, type=refnum<notifier> refnum ("notifier out"), Variant=w470) -> (data=w469:refnum<notifier>, error out=w466:errorcluster)
                      n136 = property class="VI"(reference=w462, error in=w466) -> (error out=w465:errorcluster, "Front Panel.PanelBounds"=w461:T6)  [unwired: 1 out]
                      n137 = Send Notification(notification=w461, notifier=w469, error in (no error)=w465) -> (error out=w464:errorcluster)  [unwired: 1 out]
                    }
                    frame "Get Resizable" {
                      n138 = Variant To Data(error in=w474, type=refnum<notifier> refnum ("notifier out"), Variant=w481) -> (data=w480:refnum<notifier>, error out=w477:errorcluster)
                      n139 = property class="VI"(reference=w473, error in=w477) -> (error out=w476:errorcluster, "Front Panel.Resizeable"=w472:bool)  [unwired: 1 out]
                      n140 = Send Notification(notification=w472, notifier=w480, error in (no error)=w476) -> (error out=w475:errorcluster)  [unwired: 1 out]
                    }
                    frame "Get Run VI Transparently" {
                      n141 = Variant To Data(error in=w485, type=refnum<notifier> refnum ("notifier out"), Variant=w492) -> (data=w491:refnum<notifier>, error out=w488:errorcluster)
                      n142 = property class="VI"(reference=w484, error in=w488) -> (error out=w487:errorcluster, "FP:RunTransparently"=w483:bool)  [unwired: 1 out]
                      n143 = Send Notification(notification=w483, notifier=w491, error in (no error)=w487) -> (error out=w486:errorcluster)  [unwired: 1 out]
                    }
                    frame "Get Show Menu Bar" {
                      n144 = Variant To Data(error in=w496, type=refnum<notifier> refnum ("notifier out"), Variant=w503) -> (data=w502:refnum<notifier>, error out=w499:errorcluster)
                      n145 = property class="VI"(reference=w495, error in=w499) -> (error out=w498:errorcluster, "Front Panel.ShowMenuBar"=w494:bool)  [unwired: 1 out]
                      n146 = Send Notification(notification=w494, notifier=w502, error in (no error)=w498) -> (error out=w497:errorcluster)  [unwired: 1 out]
                    }
                    frame "Get State" {
                      n147 = Variant To Data(error in=w507, type=refnum<notifier> refnum ("notifier out"), Variant=w514) -> (data=w513:refnum<notifier>, error out=w510:errorcluster)
                      n148 = property class="VI"(reference=w506, error in=w510) -> (error out=w509:errorcluster, "FP.State"=w505:T2)  [unwired: 1 out]
                      n149 = Send Notification(notification=w505, notifier=w513, error in (no error)=w509) -> (error out=w508:errorcluster)  [unwired: 1 out]
                    }
                    frame "Get Title" {
                      n150 = Variant To Data(error in=w518, type=refnum<notifier> refnum ("notifier out"), Variant=w525) -> (data=w524:refnum<notifier>, error out=w521:errorcluster)
                      n151 = property class="VI"(reference=w517, error in=w521) -> (error out=w520:errorcluster, "Front Panel.Title"=w516:string)  [unwired: 1 out]
                      n152 = Send Notification(notification=w516, notifier=w524, error in (no error)=w520) -> (error out=w519:errorcluster)  [unwired: 1 out]
                    }
                    frame "Get Title Bar Visible" {
                      n153 = Variant To Data(error in=w529, type=refnum<notifier> refnum ("notifier out"), Variant=w536) -> (data=w535:refnum<notifier>, error out=w532:errorcluster)
                      n154 = property class="VI"(reference=w528, error in=w532) -> (error out=w531:errorcluster, "Front Panel.TitleBarVis"=w527:bool)  [unwired: 1 out]
                      n155 = Send Notification(notification=w527, notifier=w535, error in (no error)=w531) -> (error out=w530:errorcluster)  [unwired: 1 out]
                    }
                    frame "Get Title Bar Colors" {
                      n156 = Variant To Data(error in=w541, type=refnum<notifier> refnum ("notifier out"), Variant=w546) -> (data=w545:refnum<notifier>, error out=w539:errorcluster)
                      n157 = property on="TitleBar" class="Bool (strict)"(error in=w539) -> (error out=w538:errorcluster, "Colors [4]"=w540:cluster{u32, u32}[])  [unwired: 1 in, 1 out]
                      n158 = Send Notification(notification=w540, notifier=w545, error in (no error)=w538) -> (error out=w542:errorcluster)  [unwired: 1 out]
                    }
                    frame "Get Transparancy" {
                      n159 = Variant To Data(error in=w550, type=refnum<notifier> refnum ("notifier out"), Variant=w557) -> (data=w556:refnum<notifier>, error out=w553:errorcluster)
                      n160 = property class="VI"(reference=w549, error in=w553) -> (error out=w552:errorcluster, "FP:Transparency"=w548:u8)  [unwired: 1 out]
                      n161 = Send Notification(notification=w548, notifier=w556, error in (no error)=w552) -> (error out=w551:errorcluster)  [unwired: 1 out]
                    }
                    frame "Get Window Bounds" {
                      n162 = Variant To Data(error in=w561, type=refnum<notifier> refnum ("notifier out"), Variant=w568) -> (data=w567:refnum<notifier>, error out=w564:errorcluster)
                      n163 = property class="VI"(reference=w560, error in=w564) -> (error out=w563:errorcluster, "Front Panel.WinBounds"=w559:T6)  [unwired: 1 out]
                      n164 = Send Notification(notification=w559, notifier=w567, error in (no error)=w563) -> (error out=w562:errorcluster)  [unwired: 1 out]
                    }
                    frame "--" {
                      # "Do Nothing Separator Only"
                    }
                    frame "Center" {
                      n165 = invoke class="VI" method="FP.Center"(error in=w573) -> (error out=w574:errorcluster)  [unwired: 2 in, 2 out]
                    }
                    frame "Close" {
                      n166 = property class="VI"(reference=w579, error in=w581) -> (reference out=w578:refnum<vi>, error out=w580:errorcluster, "FP.State"=w577:T2)
                      n167 = case shown="\"Closed\"" w577 {
                        tunnel: [w584 w587] -> w582
                        tunnel: w580 -> [w584 w586]
                        tunnel: w578 -> [_ w585]
                        frame "Closed" {
                        }
                        frame Default {
                          n168 = invoke class="VI" method="FP.Close"(reference=w585, error in=w586) -> (error out=w587:errorcluster)  [unwired: 1 in, 2 out]
                        }
                      }
                    }
                    frame "Open" {
                      n169 = Variant To Data(error in=w594, type=T7 {"Activate?"=FALSE, "State"=enum."Invalid"}, Variant=w600) -> (data=w599:T7, error out=w596:errorcluster)
                      n170 = Unbundle By Name(w599) -> ("Activate?"=w597:bool, "State"=w592:T2)
                      n171 = case shown="Default" w592 {
                        selector: w592 -> [_ w605 _]
                        tunnel: w597 -> [_ w606 _]
                        tunnel: w596 -> [w601 w604 w609]
                        tunnel: [w601 w603 w608] -> w595
                        tunnel: w593 -> [_ w602 w607]
                        frame "Invalid" {
                        }
                        frame Default {
                          n172 = invoke class="VI" method="FP.Open"(reference=w602, error in=w604, "Activate"=w606, "State"=w605) -> (error out=w603:errorcluster)  [unwired: 1 in, 4 out]
                        }
                        frame "Closed" {
                          n173 = invoke class="VI" method="FP.Close"(reference=w607, error in=w609) -> (error out=w608:errorcluster)  [unwired: 1 in, 2 out]
                        }
                      }
                      n174 = call "SendNotification.vi"("error in (no error)"=w595, "ByRefClass in"=w589) -> ("error out"=w590:errorcluster, "ByRefClass out"=w588:refnum<class "WindowFrame.lvclass">)  [unwired: 8 in]
                    }
                    frame "Run-Time Position:Centered" {
                      n175 = Variant To Data(error in=w613, type=T8 {"Monitor"=0, "Size"={"Height"=0, "Width"=0}}, Variant=w620) -> (data=w618:T8, error out=w615:errorcluster)
                      n176 = Unbundle By Name(w618) -> ("Monitor"=w612:i16, "Size"=w617:cluster{"Height":i16, "Width":i16})
                      n177 = case shown="Default" w612 {
                        selector: w612 -> [w626 _]
                        tunnel: w617 -> [w623 w638]
                        tunnel: w615 -> [w625 w640]
                        tunnel: [w624 w639] -> w614
                        tunnel: w611 -> [w621 w636]
                        frame 1.. {
                          n178 = Unbundle(w623) -> ("Height"=w622:i16)  [unwired: 1 out]
                          n179 = case shown="Default" w622 {
                            tunnel: w626 -> [w631 w635]
                            tunnel: w623 -> [w630 _]
                            tunnel: w625 -> [w629 w634]
                            tunnel: [w628 w633] -> w624
                            tunnel: w621 -> [w627 w632]
                            frame 1.. {
                              n180 = invoke class="VI" method="FP.Run-Time Position.Centered"(reference=w627, error in=w629, "Monitor"=w631, "Monitor"=w630) -> (error out=w628:errorcluster)  [unwired: 1 in, 4 out]
                            }
                            frame Default {
                              n181 = invoke class="VI" method="FP.Run-Time Position.Centered"(reference=w632, error in=w634, "Monitor"=w635) -> (error out=w633:errorcluster)  [unwired: 2 in, 4 out]
                            }
                          }
                        }
                        frame Default {
                          n182 = Unbundle(w638) -> ("Height"=w637:i16)  [unwired: 1 out]
                          n183 = case shown="1.." w637 {
                            tunnel: w638 -> [w644 _]
                            tunnel: w640 -> [w643 w647]
                            tunnel: [w642 w646] -> w639
                            tunnel: w636 -> [w641 w645]
                            frame 1.. {
                              n184 = invoke class="VI" method="FP.Run-Time Position.Centered"(reference=w641, error in=w643, "Monitor"=w644) -> (error out=w642:errorcluster)  [unwired: 2 in, 4 out]
                            }
                            frame Default {
                              n185 = invoke class="VI" method="FP.Run-Time Position.Centered"(reference=w645, error in=w647) -> (error out=w646:errorcluster)  [unwired: 3 in, 4 out]
                            }
                          }
                        }
                      }
                    }
                    frame "Run-Time Position:Custom" {
                      n186 = Variant To Data(error in=w650, type=T9 {"Position"={"Top"=0, "Left"=0}, "Size"={"Height"=0, "Width"=0}}, Variant=w658) -> (data=w656:T9, error out=w652:errorcluster)
                      n187 = Unbundle By Name(w656) -> ("Position"=w655:cluster{"Top":i16, "Left":i16}, "Size"=w654:cluster{"Height":i16, "Width":i16})
                      n188 = invoke class="VI" method="FP.Run-Time Position.Custom"(reference=w649, error in=w652, "Size"=w655, "Position"=w654) -> (error out=w651:errorcluster)  [unwired: 1 in, 4 out]
                    }
                    frame "Run-Time Position:Get Position" {
                      n189 = Variant To Data(error in=w660, type=refnum<notifier> refnum ("notifier out"), Variant=w668) -> (data=w667:refnum<notifier>, error out=w663:errorcluster)
                      n190 = invoke class="VI" method="FP.Run-Time Pos.Get"(error in=w663) -> (error out=w662:errorcluster, "type"=w675:T16, "top"=w674:cluster{"Top":i16, "Left":i16}, "left"=w673:cluster{"Height":i16, "Width":i16}, "width"=w672:i16, "height"=w671:bool, "monitor"=w670:bool)  [unwired: 8 in, 2 out]
                      n191 = Bundle By Name(cluster=T10 {"Type"=enum."Unchanged", "Position"={"Top"=0, "Left"=0}, "Size"={"Height"=0, "Width"=0}, "Monitor"=0, "Use Current Position"=FALSE, "Use Current Size"=FALSE}, "Type"=w675, "Position"=w674, "Size"=w673, "Monitor"=w672, "Use Current Position"=w671, "Use Current Size"=w670) -> (w669:T10)
                      n192 = Send Notification(notification=w669, notifier=w667, error in (no error)=w662) -> (error out=w661:errorcluster)  [unwired: 1 out]
                    }
                    frame "Run-Time Position:Maximized" {
                      n193 = Variant To Data(error in=w679, type=i16 0 ("Monitor"), Variant=w684) -> (data=w683:i16, error out=w681:errorcluster)
                      n194 = invoke class="VI" method="FP.Run-Time Position.Maximized"(reference=w677, error in=w681, "Monitor"=w683) -> (error out=w680:errorcluster)  [unwired: 1 in, 3 out]
                    }
                    frame "Run-Time Position:Minimized" {
                      n195 = Variant To Data(error in=w688, type=i16 0 ("Monitor"), Variant=w693) -> (data=w692:i16, error out=w690:errorcluster)
                      n196 = invoke class="VI" method="FP.Run-Time Position.Minimized"(reference=w686, error in=w690, "Monitor"=w692) -> (error out=w689:errorcluster)  [unwired: 1 in, 3 out]
                    }
                    frame "Run-Time Position:Unchanged" {
                      n197 = invoke class="VI" method="FP.Run-Time Pos.Unchanged"(reference=w695, error in=w696) -> (error out=w697:errorcluster)  [unwired: 1 in, 2 out]
                    }
                    frame "---" {
                      # "Do Nothing Separator Only"
                    }
                    frame "Insert VI" {
                      n198 = Variant To Data(error in=w708, type=w702, Variant=w707) -> (data=w704:refnum<vi>, error out=w706:errorcluster)
                      n199 = invoke on="MainSubPanel" class="SubPnl" method="Insert VI"(error in=w706, "VI Ref"=w704) -> (error out=w705:errorcluster)  [unwired: 2 in, 3 out]
                    }
                    frame "Insert VI Index" {
                      n200 = Variant To Data(error in=w723, type=T11 {"Z-Order"=0, "Position"={"Left"=0, "Top"=0}, "Size"={"Width"=0, "Height"=0}, "VI Ref"=refnum}, Variant=w722) -> (data=w720:T11, error out=w718:errorcluster)
                      n201 = Unbundle By Name(w720) -> ("Z-Order"=w719:i32, "Position"=w714:T12, "Size"=w713:T13, "VI Ref"=w712:refnum<vi>)
                      n202 = Index Array(array=w710, index=w719) -> (element=w715:refnum<vi>)
                      n203 = property class="SubPnl"(reference=w715, error in=w718, "Position"=w714, "Container Bounds"=w713) -> (reference out=w711:refnum<vi>, error out=w717:errorcluster)
                      n204 = invoke on="Invoke Node" class="SubPnl" method="Insert VI"(reference=w711, error in=w717, "VI Ref"=w712) -> (error out=w716:errorcluster)  [unwired: 1 in, 3 out]
                    }
                    frame "Remove VI Index" {
                      n205 = Variant To Data(error in=w736, type=0, Variant=w735) -> (data=w726:i32, error out=w734:errorcluster)
                      n206 = Index Array(array=w725, index=w726) -> (element=w731:refnum<vi>)
                      n207 = property class="SubPnl"(reference=w731, error in=w734, "Position"=T12 {"Left"=-10, "Top"=-10}, "Container Bounds"=T13 {"Width"=5, "Height"=5}) -> (reference out=w730:refnum<vi>, error out=w733:errorcluster)
                      n208 = invoke on="Invoke Node" class="SubPnl" method="Remove VI"(reference=w730, error in=w733) -> (error out=w732:errorcluster)  [unwired: 1 in, 2 out]
                    }
                    frame "Remove VI" {
                      n209 = invoke on="MainSubPanel" class="SubPnl" method="Remove VI"(error in=w740) -> (error out=w739:errorcluster)  [unwired: 2 in, 2 out]
                    }
                    frame "Exit" {
                    }
                  }
                }
                event Pane Size {
                  n210 = event-data() -> ("PaneRef"=w749:refnum<vi>)  [unwired: 1 in]
                  n211 = property class="Pane"(reference=w749) -> ("Bounds"=w747:T13)  [unwired: 1 in, 2 out]
                  n212 = property on="MainSubPanel" class="SubPnl"("Position"=T12 {"Left"=0, "Top"=0}, "Container Bounds"=w747) -> ()  [unwired: 2 in, 2 out]
                }
                event Panel Close? {
                  w754 = FALSE ("Discard?")
                  n213 = event-data() -> ()  [unwired: 1 in, 1 out]
                  n214 = event-data("Discard?"=w754) -> ()  [unwired: 1 in, 1 out]
                }
                event VI Activation {
                  w770 = T4."Disabled and Grayed Out" ("Disabled")
                  w771 = T4."Enabled" ("Disabled")
                  n215 = event-data() -> ()  [unwired: 1 in, 7 out]
                  n216 = local write "TitleBar"(TRUE ("TitleBar")) -> ()
                  n217 = property class="VI"(reference=w757, error in=w758) -> (error out=w762:errorcluster, "Front Panel.Minimizeable"=w769:bool, "Front Panel.Resizeable"=w768:bool, "Front Panel.Closeable"=w767:bool)  [unwired: 1 out]
                  n218 = Select(t=w771, s=w769, f=w770) -> (s? t:f=w766:T4)
                  n219 = Select(t=w771, s=w768, f=w770) -> (s? t:f=w765:T4)
                  n220 = Select(t=w771, s=w767, f=w770) -> (s? t:f=w764:T4)
                  n221 = property on="Minimize" class="Bool"(error in=w762, "DisabledEnum"=w766) -> (error out=w761:errorcluster)  [unwired: 1 in, 1 out]
                  n222 = property on="Maximize" class="Bool"(error in=w761, "DisabledEnum"=w765) -> (error out=w760:errorcluster)  [unwired: 1 in, 1 out]
                  n223 = property on="Close" class="Bool"(error in=w760, "DisabledEnum"=w764) -> (error out=w759:errorcluster)  [unwired: 1 in, 1 out]
                }
                event event #0x53 {
                  n224 = event-data() -> ()  [unwired: 1 in, 7 out]
                  n225 = local write "TitleBar"(FALSE ("TitleBar")) -> ()
                  n226 = property on="Minimize" class="Bool"("DisabledEnum"=T4."Disabled and Grayed Out" ("Disabled")) -> ()  [unwired: 2 in, 2 out]
                }
              }
            }
            frame Error {
              n227 = call <vilib>:"Simple Error Handler.vi"("error in (no error)"=w783) -> ("error out"=w782:errorcluster)  [unwired: 4 in, 4 out]
              n228 = call <vilib>:"Clear Errors.vi"("error in (no error)"=w782) -> ("error out"=w781:errorcluster)  [unwired: 5 in, 1 out]
            }
          }
        }
      }
      frame "Close" {
        n229 = Close Reference(reference=w787, error in (no error)=w789) -> (error out=w788:errorcluster)
        n230 = Unregister For Events(event registration refnum=w790, error in=w788) -> (error out=w791:errorcluster)
        n231 = call "SendNotification.vi"("error in (no error)"=w791, "ByRefClass in"=w784) -> ("error out"=w786:errorcluster, "ByRefClass out"=w785:refnum<class "WindowFrame.lvclass">)  [unwired: 8 in]
      }
    }
  }
  "error out" <- w3
  "WindowFrame out" <- w7
